vi "rsscope_core_global.vi"() -> ()   [LabVIEW 2014] (continued)
trigger search. The state search is a qualified edge search. The state search is only available for analog channel sources (Ch1 to Ch4)."}, {"Level"=4, "Class Only"=FALSE, "Identifier"="RSSCOPE_ATTR_SEARCH_TRIGGER_STATE_ENABLED", "Descriptive Name"="Search Trigger State Enabled", "Data Type"=3, "Command"="SEAR:TRIG:STAT", "Access"=2, "Range Table"="", "Read Callback"="rsscope_FormatSearchNameBoolean_ReadCallback.vi", "Write Callback"="rsscope_FormatSearchNameBoolean_WriteCallback.vi", "Supported Models"="", "Instrument Options"="", "Flags"=0, "Help"="Includes the search conditions for the state trigger event type in the next search.\n\nAvailable Repeated Capabilities:\nNone\n\nRemote-control command(s):\nSEARch:TRIGger:STATe[:STATe]"}, {"Level"=4, "Class Only"=FALSE, "Identifier"="RSSCOPE_ATTR_SEARCH_TRIGGER_STATE_CLOCK_SOURCE", "Descriptive Name"="Search Trigger State Clock Source", "Data Type"=0, "Command"="SEAR:TRIG:STAT:CSO", "Access"=2, "Range Table"="RsScope_rngSearchTriggerStateClockSource", "Read Callback"="rsscope_FormatSearchNameInt32_ReadCallback.vi", "Write Callback"="rsscope_FormatSearchNameInt32_WriteCallback.vi", "Supported Models"="", "Instrument Options"="", "Flags"=0, "Help"="Sets the source of the clock signal.\n\nAvailable Repeated Capabilities:\nNone\n\nRemote-control command(s):\nSEARch:TRIGger:STATe:CSOurce"}, {"Level"=4, "Class Only"=FALSE, "Identifier"="RSSCOPE_ATTR_SEARCH_TRIGGER_STATE_LEVEL", "Descriptive Name"="Search Trigger State Level", "Data Type"=1, "Command"="SEAR:TRIG:STAT:CLEV", "Access"=2, "Range Table"="RsScope_rngSearchTriggerClockLevel", "Read Callback"="rsscope_FormatSearchNameReal64_ReadCallback.vi", "Write Callback"="rsscope_FormatSearchNameReal64_WriteCallback.vi", "Supported Models"="", "Instrument Options"="", "Flags"=0, "Help"="Sets the trigger level of the clock signal.\n\nAvailable Repeated Capabilities:\nNone\n\nRemote-control command(s):\nSEARch:TRIGger:STATe:CLEVel"}, {"Level"=4, "Class Only"=FALSE, "Identifier"="RSSCOPE_ATTR_SEARCH_TRIGGER_STATE_CLOCK_EDGE", "Descriptive Name"="Search Trigger State Clock Edge", "Data Type"=0, "Command"="SEAR:TRIG:STAT:CEDG", "Access"=2, "Range Table"="rsscope_rngTriggerSlope", "Read Callback"="rsscope_FormatSearchNameInt32_ReadCallback.vi", "Write Callback"="rsscope_FormatSearchNameInt32_WriteCallback.vi", "Supported Models"="", "Instrument Options"="", "Flags"=0, "Help"="Sets the trigger edge of the clock signal.\n\nAvailable Repeated Capabilities:\nNone\n\nRemote-control command(s):\nSEARch:TRIGger:STATe:CEDGe"}, {"Level"=4, "Class Only"=FALSE, "Identifier"="RSSCOPE_ATTR_SEARCH_TRIGGER_STATE_COPY_FROM_A", "Descriptive Name"="Search Trigger State Copy From A", "Data Type"=4, "Command"="SEAR:TRIG:STAT:ACOP", "Access"=1, "Range Table"="", "Read Callback"="", "Write Callback"="rsscope_FormatSearchNameEvent_WriteCallback.vi", "Supported Models"="", "Instrument Options"="", "Flags"=0, "Help"="Copies the trigger event configuration from Trigger A for the selected channel source to the search condition settings. Set the selected search name with RSSCOPE_ATTR_SELECTED_SEARCH_NAME.\n\nAvailable Repeated Capabilities:\nNone\n\nRemote-control command(s):\nSEARch:TRIGger:STATe:ACOPy"}, {"Level"=4, "Class Only"=TRUE, "Identifier"="", "Descriptive Name"="Trigger Qualification", "Data Type"=0, "Command"="", "Access"=0, "Range Table"="", "Read Callback"="", "Write Callback"="", "Supported Models"="", "Instrument Options"="", "Flags"=0, "Help"="By qualifying a trigger event, you can logically combine the trigger signal with the state of other digital channel signals.\nThe instrument triggers if both of the following apply:\n- The basic conditions of the trigger event definition are fulfilled.\n- The logical conditions of the trigger qualification are true.\n\nQualification is not supported with slew rate, Data2Clock, and serial pattern trigger types.\n\nThe A-event and B-event in a trigger sequence can have their own trigger qualification. Qualification is not available for R-events (Suffix m = 3).\n\nExample: Trigger on write access of a specific device of a bus system In circuits using SPI, several slave devices use the same lines for reading and writing data, and each slave has its own select line. To trigger on write access of specific slave, the write line is the trigger source and the select line of the slave is set as qualifiying."}, {"Level"=5, "Class Only"=FALSE, "Identifier"="RSSCOPE_ATTR_SEARCH_STATE_TRIGGER_QUALIFICATION_ENABLED_CHANNEL_1", "Descriptive Name"="Search State Trigger Qualification Enabled Channel 1", "Data Type"=3, "Command"="SEAR:TRIG:STAT:A", "Access"=2, "Range Table"="", "Read Callback"="rsscope_FormatSearchNameBoolean_ReadCallback.vi", "Write Callback"="rsscope_FormatSearchNameBoolean_WriteCallback.vi", "Supported Models"="", "Instrument Options"="", "Flags"=0, "Help"="Enables the channel to be considered in the state search. You can enable all channel signals except for the trigger source. Digital channels are not available.\n\nAvailable Repeated Capabilities:\nNone\n\nRemote-control command(s):\nSEARch:TRIGger:STATe:A[:ENABle]"}, {"Level"=5, "Class Only"=FALSE, "Identifier"="RSSCOPE_ATTR_SEARCH_STATE_TRIGGER_QUALIFICATION_ENABLED_CHANNEL_2", "Descriptive Name"="Search State Trigger Qualification Enabled Channel 2", "Data Type"=3, "Command"="SEAR:TRIG:STAT:B", "Access"=2, "Range Table"="", "Read Callback"="rsscope_FormatSearchNameBoolean_ReadCallback.vi", "Write Callback"="rsscope_FormatSearchNameBoolean_WriteCallback.vi", "Supported Models"="", "Instrument Options"="", "Flags"=0, "Help"="Enables the channel to be considered in the state search. You can enable all channel signals except for the trigger source. Digital channels are not available.\n\nAvailable Repeated Capabilities:\nNone\n\nRemote-control command(s):\nSEARch:TRIGger:STATe:B[:ENABle]"}, {"Level"=5, "Class Only"=FALSE, "Identifier"="RSSCOPE_ATTR_SEARCH_STATE_TRIGGER_QUALIFICATION_ENABLED_CHANNEL_3", "Descriptive Name"="Search State Trigger Qualification Enabled Channel 3", "Data Type"=3, "Command"="SEAR:TRIG:STAT:C", "Access"=2, "Range Table"="", "Read Callback"="rsscope_FormatSearchNameBoolean_ReadCallback.vi", "Write Callback"="rsscope_FormatSearchNameBoolean_WriteCallback.vi", "Supported Models"="", "Instrument Options"="", "Flags"=0, "Help"="Enables the channel to be considered in the state search. You can enable all channel signals except for the trigger source. Digital channels are not available.\n\nAvailable Repeated Capabilities:\nNone\n\nRemote-control command(s):\nSEARch:TRIGger:STATe:C[:ENABle]"}, {"Level"=5, "Class Only"=FALSE, "Identifier"="RSSCOPE_ATTR_SEARCH_STATE_TRIGGER_QUALIFICATION_ENABLED_CHANNEL_4", "Descriptive Name"="Search State Trigger Qualification Enabled Channel 4", "Data Type"=3, "Command"="SEAR:TRIG:STAT:D", "Access"=2, "Range Table"="", "Read Callback"="rsscope_FormatSearchNameBoolean_ReadCallback.vi", "Write Callback"="rsscope_FormatSearchNameBoolean_WriteCallback.vi", "Supported Models"="", "Instrument Options"="", "Flags"=0, "Help"="Enables the channel to be considered in the state search. You can enable all channel signals except for the trigger source. Digital channels are not available.\n\nAvailable Repeated Capabilities:\nNone\n\nRemote-control command(s):\nSEARch:TRIGger:STATe:D[:ENABle]"}, {"Level"=5, "Class Only"=FALSE, "Identifier"="RSSCOPE_ATTR_SEARCH_STATE_TRIGGER_QUALIFICATION_LOGIC_CHANNEL_1", "Descriptive Name"="Search State Trigger Qualification Logic Channel 1", "Data Type"=0, "Command"="SEAR:TRIG:STAT:A:LOG", "Access"=2, "Range Table"="rsscope_rngTriggerQualificationLogic", "Read Callback"="rsscope_FormatSearchNameInt32_ReadCallback.vi", "Write Callback"="rsscope_FormatSearchNameInt32_WriteCallback.vi", "Supported Models"="", "Instrument Options"="", "Flags"=0, "Help"="Defines the logic for the indicated channel.\n\nAvailable Repeated Capabilities:\nNone\n\nRemote-control command(s):\nSEARch:TRIGger:STATe:A:LOGic"}, {"Level"=5, "Class Only"=FALSE, "Identifier"="RSSCOPE_ATTR_SEARCH_STATE_TRIGGER_QUALIFICATION_LOGIC_CHANNEL_2", "Descriptive Name"="Search State Trigger Qualification Logic Channel 2", "Data Type"=0, "Command"="SEAR:TRIG:STAT:B:LOG", "Access"=2, "Range Table"="rsscope_rngTriggerQualificationLogic", "Read Callback"="rsscope_FormatSearchNameInt32_ReadCallback.vi", "Write Callback"="rsscope_FormatSearchNameInt32_WriteCallback.vi", "Supported Models"="", "Instrument Options"="", "Flags"=0, "Help"="Defines the logic for the indicated channel.\n\nAvailable Repeated Capabilities:\nNone\n\nRemote-control command(s):\nSEARch:TRIGger:STATe:B:LOGic"}, {"Level"=5, "Class Only"=FALSE, "Identifier"="RSSCOPE_ATTR_SEARCH_STATE_TRIGGER_QUALIFICATION_LOGIC_CHANNEL_3", "Descriptive Name"="Search State Trigger Qualification Logic Channel 3", "Data Type"=0, "Command"="SEAR:TRIG:STAT:C:LOG", "Access"=2, "Range Table"="rsscope_rngTriggerQualificationLogic", "Read Callback"="rsscope_FormatSearchNameInt32_ReadCallback.vi", "Write Callback"="rsscope_FormatSearchNameInt32_WriteCallback.vi", "Supported Models"="", "Instrument Options"="", "Flags"=0, "Help"="Defines the logic for the indicated channel.\n\nAvailable Repeated Capabilities:\nNone\n\nRemote-control command(s):\nSEARch:TRIGger:STATe:C:LOGic"}, {"Level"=5, "Class Only"=FALSE, "Identifier"="RSSCOPE_ATTR_SEARCH_STATE_TRIGGER_QUALIFICATION_LOGIC_CHANNEL_4", "Descriptive Name"="Search State Trigger Qualification Logic Channel 4", "Data Type"=0, "Command"="SEAR:TRIG:STAT:D:LOG", "Access"=2, "Range Table"="rsscope_rngTriggerQualificationLogic", "Read Callback"="rsscope_FormatSearchNameInt32_ReadCallback.vi", "Write Callback"="rsscope_FormatSearchNameInt32_WriteCallback.vi", "Supported Models"="", "Instrument Options"="", "Flags"=0, "Help"="Defines the logic for the indicated channel.\n\nAvailable Repeated Capabilities:\nNone\n\nRemote-control command(s):\nSEARch:TRIGger:STATe:D:LOGic"}, {"Level"=5, "Class Only"=FALSE, "Identifier"="RSSCOPE_ATTR_SEARCH_STATE_TRIGGER_QUALIFICATION_LOGIC_CHANNELS_1_2", "Descriptive Name"="Search State Trigger Qualification Logic Channels 1 2", "Data Type"=0, "Command"="SEAR:TRIG:STAT:AB:LOG", "Access"=2, "Range Table"="rsscope_rngLogic", "Read Callback"="rsscope_FormatSearchNameInt32_ReadCallback.vi", "Write Callback"="rsscope_FormatSearchNameInt32_WriteCallback.vi", "Supported Models"="", "Instrument Options"="", "Flags"=0, "Help"="Defines the logical combination of the indicated channels after evaluating the previous logical operations.\n\nAvailable Repeated Capabilities:\nNone\n\nRemote-control command(s):\nSEARch:TRIGger:STATe:AB:LOGic"}, {"Level"=5, "Class Only"=FALSE, "Identifier"="RSSCOPE_ATTR_SEARCH_STATE_TRIGGER_QUALIFICATION_LOGIC_CHANNELS_3_4", "Descriptive Name"="Search State Trigger Qualification Logic Channels 3 4", "Data Type"=0, "Command"="SEAR:TRIG:STAT:CD:LOG", "Access"=2, "Range Table"="rsscope_rngLogic", "Read Callback"="rsscope_FormatSearchNameInt32_ReadCallback.vi", "Write Callback"="rsscope_FormatSearchNameInt32_WriteCallback.vi", "Supported Models"="", "Instrument Options"="", "Flags"=0, "Help"="Defines the logical combination of the indicated channels after evaluating the previous logical operations.\n\nAvailable Repeated Capabilities:\nNone\n\nRemote-control command(s):\nSEARch:TRIGger:STATe:CD:LOGic"}, {"Level"=5, "Class Only"=FALSE, "Identifier"="RSSCOPE_ATTR_SEARCH_STATE_TRIGGER_QUALIFICATION_LOGIC_CHANNELS_ALL", "Descriptive Name"="Search State Trigger Qualification Logic Channels All", "Data Type"=0, "Command"="SEAR:TRIG:STAT:ABCD:LOG", "Access"=2, "Range Table"="rsscope_rngLogic", "Read Callback"="rsscope_FormatSearchNameInt32_ReadCallback.vi", "Write Callback"="rsscope_FormatSearchNameInt32_WriteCallback.vi", "Supported Models"="", "Instrument Options"="", "Flags"=0, "Help"="Defines the logical combination of the indicated channels after evaluating the result of channels 1+2 and 3+4.\n\nAvailable Repeated Capabilities:\nNone\n\nRemote-control command(s):\nSEARch:TRIGger:STATe:ABCD:LOGic"}, {"Level"=3, "Class Only"=TRUE, "Identifier"="", "Descriptive Name"="Pattern", "Data Type"=0, "Command"="", "Access"=0, "Range Table"="", "Read Callback"="", "Write Callback"="", "Supported Models"="", "Instrument Options"="", "Flags"=0, "Help"="This class configures the conditions for the pattern trigger search."}, {"Level"=4, "Class Only"=FALSE, "Identifier"="RSSCOPE_ATTR_SEARCH_TRIGGER_PATTERN_ENABLED", "Descriptive Name"="Search Trigger Pattern Enabled", "Data Type"=3, "Command"="SEAR:TRIG:PATT", "Access"=2, "Range Table"="", "Read Callback"="rsscope_FormatSearchNameBoolean_ReadCallback.vi", "Write Callback"="rsscope_FormatSearchNameBoolean_WriteCallback.vi", "Supported Models"="", "Instrument Options"="", "Flags"=0, "Help"="Includes the search conditions for the pattern trigger event type in the next search.\n\nAvailable Repeated Capabilities:\nNone\n\nRemote-control command(s):\nSEARch:TRIGger:PATTern[:STATe]"}, {"Level"=4, "Class Only"=FALSE, "Identifier"="RSSCOPE_ATTR_SEARCH_TRIGGER_PATTERN_MODE", "Descriptive Name"="Search Trigger Pattern Mode", "Data Type"=0, "Command"="SEAR:TRIG:PATT:MODE", "Access"=2, "Range Table"="RsScope_rngSearchTriggerPatternMode", "Read Callback"="rsscope_FormatSearchNameInt32_ReadCallback.vi", "Write Callback"="rsscope_FormatSearchNameInt32_WriteCallback.vi", "Supported Models"="", "Instrument Options"="", "Flags"=0, "Help"="Adds additional time limitation to the pattern definition.\n\nAvailable Repeated Capabilities:\nNone\n\nRemote-control command(s):\nSEARch:TRIGger:PATTern:MODE"}, {"Level"=4, "Class Only"=FALSE, "Identifier"="RSSCOPE_ATTR_SEARCH_TRIGGER_PATTERN_TIMEOUT_CONDITION", "Descriptive Name"="Search Trigger Pattern Timeout Condition", "Data Type"=0, "Command"="SEAR:TRIG:PATT:TIM:MODE", "Access"=2, "Range Table"="RsScope_rngSearchTriggerPatternTimeoutMode", "Read Callback"="rsscope_FormatSearchNameInt32_ReadCallback.vi", "Write Callback"="rsscope_FormatSearchNameInt32_WriteCallback.vi", "Supported Models"="", "Instrument Options"="", "Flags"=0, "Help"="Defines the condition for the timeout.\n\nAvailable Repeated Capabilities:\nNone\n\nRemote-control command(s):\nSEARch:TRIGger:PATTern:TIMeout:MODE"}, {"Level"=4, "Class Only"=FALSE, "Identifier"="RSSCOPE_ATTR_SEARCH_TRIGGER_PATTERN_TIMEOUT", "Descriptive Name"="Search Trigger Pattern Timeout", "Data Type"=1, "Command"="SEAR:TRIG:PATT:TIM", "Access"=2, "Range Table"="RsScope_rngSearchTriggerWidth", "Read Callback"="rsscope_FormatSearchNameReal64_ReadCallback.vi", "Write Callback"="rsscope_FormatSearchNameReal64_WriteCallback.vi", "Supported Models"="", "Instrument Options"="", "Flags"=0, "Help"="Defines how long the result of the pattern condition must keep the given state.\n\nAvailable Repeated Capabilities:\nNone\n\nRemote-control command(s):\nSEARch:TRIGger:PATTern:TIMeout[:TIME]"}, {"Level"=4, "Class Only"=FALSE, "Identifier"="RSSCOPE_ATTR_SEARCH_TRIGGER_PATTERN_WIDTH", "Descriptive Name"="Search Trigger Pattern Width", "Data Type"=1, "Command"="SEAR:TRIG:PATT:WIDT", "Access"=2, "Range Table"="RsScope_rngSearchTriggerWidth", "Read Callback"="rsscope_FormatSearchNameReal64_ReadCallback.vi", "Write Callback"="rsscope_FormatSearchNameReal64_WriteCallback.vi", "Supported Models"="", "Instrument Options"="", "Flags"=0, "Help"="For the ranges &apos;Within&apos; and &apos;Outside&apos;, the width defines the center of a range which is defined by the limits &apos;Delta&apos;.\nFor the ranges &apos;Shorter&apos; and &apos;Longer&apos;, the width defines the maximum and minimum pulse width, respectively.\n\nAvailable Repeated Capabilities:\nNone\n\nRemote-control command(s):\nSEARch:TRIGger:PATTern:WIDTh[:WIDTh]"}, {"Level"=4, "Class Only"=FALSE, "Identifier"="RSSCOPE_ATTR_SEARCH_TRIGGER_PATTERN_WIDTH_DELTA", "Descriptive Name"="Search Trigger Pattern Width Delta", "Data Type"=1, "Command"="SEAR:TRIG:PATT:WIDT:DELT", "Access"=2, "Range Table"="RsScope_rngSearchTriggerPatternDelta", "Read Callback"="rsscope_FormatSearchNameReal64_ReadCallback.vi", "Write Callback"="rsscope_FormatSearchNameReal64_WriteCallback.vi", "Supported Models"="", "Instrument Options"="", "Flags"=0, "Help"="For the ranges &apos;Within&apos; and &apos;Outside&apos;, the width defines the center of a range which is defined by the limits &apos;+/-Delta&apos;. For the ranges &apos;Shorter&apos; and &apos;Longer&apos;, the width defines the maximum and minimum pulse width, respectively.\n\nAvailable Repeated Capabilities:\nNone\n\nRemote-control command(s):\nSEARch:TRIGger:PATTern:WIDTh:DELTa"}, {"Level"=4, "Class Only"=FALSE, "Identifier"="RSSCOPE_ATTR_SEARCH_TRIGGER_PATTERN_WIDTH_CONDITION", "Descriptive Name"="Search Trigger Pattern Width Condition", "Data Type"=0, "Command"="SEAR:TRIG:PATT:WIDT:RANG", "Access"=2, "Range Table"="rsscope_rngWidthCondition", "Read Callback"="rsscope_FormatSearchNameInt32_ReadCallback.vi", "Write Callback"="rsscope_FormatSearchNameInt32_WriteCallback.vi", "Supported Models"="", "Instrument Options"="", "Flags"=0, "Help"="Defines how the range of a pulse width is defined for keeping up the true result of the pattern condition.\n\nAvailable Repeated Capabilities:\nNone\n\nRemote-control command(s):\nSEARch:TRIGger:PATTern:WIDTh:RANGe"}, {"Level"=4, "Class Only"=FALSE, "Identifier"="RSSCOPE_ATTR_SEARCH_TRIGGER_PATTERN_COPY_FROM_A", "Descriptive Name"="Search Trigger Pattern Copy From A", "Data Type"=4, "Command"="SEAR:TRIG:PATT:ACOP", "Access"=1, "Range Table"="", "Read Callback"="", "Write Callback"="rsscope_FormatSearchNameEvent_WriteCallback.vi", "Supported Models"="", "Instrument Options"="", "Flags"=0, "Help"="Copies the trigger event configuration from Trigger A for the selected channel source to the search condition settings. Set the selected search name with RSSCOPE_ATTR_SELECTED_SEARCH_NAME.\n\nAvailable Repeated Capabilities:\nNone\n\nRemote-control command(s):\nSEARch:TRIGger:PATTern:ACOPy"}, {"Level"=4, "Class Only"=TRUE, "Identifier"="", "Descriptive Name"="Trigger Qualification", "Data Type"=0, "Command"="", "Access"=0, "Range Table"="", "Read Callback"="", "Write Callback"="", "Supported Models"="", "Instrument Options"="", "Flags"=0, "Help"="By qualifying a trigger event, you can logically combine the trigger signal with the state of other digital channel signals.\nThe instrument triggers if both of the following apply:\n- The basic conditions of the trigger event definition are fulfilled.\n- The logical conditions of the trigger qualification are true.\n\nQualification is not supported with slew rate, Data2Clock, and serial pattern trigger types.\n\nThe A-event and B-event in a trigger sequence can have their own trigger qualification. Qualification is not available for R-events (Suffix m = 3).\n\nExample: Trigger on write access of a specific device of a bus system In circuits using SPI, several slave devices use the same lines for reading and writing data, and each slave has its own select line. To trigger on write access of specific slave, the write line is the trigger source and the select line of the slave is set as qualifiying."}, {"Level"=5, "Class Only"=FALSE, "Identifier"="RSSCOPE_ATTR_SEARCH_PATTERN_TRIGGER_QUALIFICATION_ENABLED_CHANNEL_1", "Descriptive Name"="Search Pattern Trigger Qualification Enabled Channel 1", "Data Type"=3, "Command"="SEAR:TRIG:PATT:A", "Access"=2, "Range Table"="", "Read Callback"="rsscope_FormatSearchNameBoolean_ReadCallback.vi", "Write Callback"="rsscope_FormatSearchNameBoolean_WriteCallback.vi", "Supported Models"="", "Instrument Options"="", "Flags"=0, "Help"="Enables the channel to be considered in the pattern search. The trigger source channel is selected by default. Digital channels are not available.\n\nAvailable Repeated Capabilities:\nNone\n\nRemote-control command(s):\nSEARch:TRIGger:PATTern:A[:ENABle]"}, {"Level"=5, "Class Only"=FALSE, "Identifier"="RSSCOPE_ATTR_SEARCH_PATTERN_TRIGGER_QUALIFICATION_ENABLED_CHANNEL_2", "Descriptive Name"="Search Pattern Trigger Qualification Enabled Channel 2", "Data Type"=3, "Command"="SEAR:TRIG:PATT:B", "Access"=2, "Range Table"="", "Read Callback"="rsscope_FormatSearchNameBoolean_ReadCallback.vi", "Write Callback"="rsscope_FormatSearchNameBoolean_WriteCallback.vi", "Supported Models"="", "Instrument Options"="", "Flags"=0, "Help"="Enables the channel to be considered in the pattern search. The trigger source channel is selected by default. Digital channels are not available.\n\nAvailable Repeated Capabilities:\nNone\n\nRemote-control command(s):\nSEARch:TRIGger:PATTern:B[:ENABle]"}, {"Level"=5, "Class Only"=FALSE, "Identifier"="RSSCOPE_ATTR_SEARCH_PATTERN_TRIGGER_QUALIFICATION_ENABLED_CHANNEL_3", "Descriptive Name"="Search Pattern Trigger Qualification Enabled Channel 3", "Data Type"=3, "Command"="SEAR:TRIG:PATT:C", "Access"=2, "Range Table"="", "Read Callback"="rsscope_FormatSearchNameBoolean_ReadCallback.vi", "Write Callback"="rsscope_FormatSearchNameBoolean_WriteCallback.vi", "Supported Models"="", "Instrument Options"="", "Flags"=0, "Help"="Enables the channel to be considered in the pattern search. The trigger source channel is selected by default. Digital channels are not available.\n\nAvailable Repeated Capabilities:\nNone\n\nRemote-control command(s):\nSEARch:TRIGger:PATTern:C[:ENABle]"}, {"Level"=5, "Class Only"=FALSE, "Identifier"="RSSCOPE_ATTR_SEARCH_PATTERN_TRIGGER_QUALIFICATION_ENABLED_CHANNEL_4", "Descriptive Name"="Search Pattern Trigger Qualification Enabled Channel 4", "Data Type"=3, "Command"="SEAR:TRIG:PATT:D", "Access"=2, "Range Table"="", "Read Callback"="rsscope_FormatSearchNameBoolean_ReadCallback.vi", "Write Callback"="rsscope_FormatSearchNameBoolean_WriteCallback.vi", "Supported Models"="", "Instrument Options"="", "Flags"=0, "Help"="Enables the channel to be considered in the pattern search. The trigger source channel is selected by default. Digital channels are not available.\n\nAvailable Repeated Capabilities:\nNone\n\nRemote-control command(s):\nSEARch:TRIGger:PATTern:D[:ENABle]"}, {"Level"=5, "Class Only"=FALSE, "Identifier"="RSSCOPE_ATTR_SEARCH_PATTERN_TRIGGER_QUALIFICATION_LOGIC_CHANNEL_1", "Descriptive Name"="Search Pattern Trigger Qualification Logic Channel 1", "Data Type"=0, "Command"="SEAR:TRIG:PATT:A:LOG", "Access"=2, "Range Table"="rsscope_rngTriggerQualificationLogic", "Read Callback"="rsscope_FormatSearchNameInt32_ReadCallback.vi", "Write Callback"="rsscope_FormatSearchNameInt32_WriteCallback.vi", "Supported Models"="", "Instrument Options"="", "Flags"=0, "Help"="Defines the logic for the indicated channel.\n\nAvailable Repeated Capabilities:\nNone\n\nRemote-control command(s):\nSEARch:TRIGger:PATTern:A:LOGic"}, {"Level"=5, "Class Only"=FALSE, "Identifier"="RSSCOPE_ATTR_SEARCH_PATTERN_TRIGGER_QUALIFICATION_LOGIC_CHANNEL_2", "Descriptive Name"="Search Pattern Trigger Qualification Logic Channel 2", "Data Type"=0, "Command"="SEAR:TRIG:PATT:B:LOG", "Access"=2, "Range Table"="rsscope_rngTriggerQualificationLogic", "Read Callback"="rsscope_FormatSearchNameInt32_ReadCallback.vi", "Write Callback"="rsscope_FormatSearchNameInt32_WriteCallback.vi", "Supported Models"="", "Instrument Options"="", "Flags"=0, "Help"="Defines the logic for the indicated channel.\n\nAvailable Repeated Capabilities:\nNone\n\nRemote-control command(s):\nSEARch:TRIGger:PATTern:B:LOGic"}, {"Level"=5, "Class Only"=FALSE, "Identifier"="RSSCOPE_ATTR_SEARCH_PATTERN_TRIGGER_QUALIFICATION_LOGIC_CHANNEL_3", "Descriptive Name"="Search Pattern Trigger Qualification Logic Channel 3", "Data Type"=0, "Command"="SEAR:TRIG:PATT:C:LOG", "Access"=2, "Range Table"="rsscope_rngTriggerQualificationLogic", "Read Callback"="rsscope_FormatSearchNameInt32_ReadCallback.vi", "Write Callback"="rsscope_FormatSearchNameInt32_WriteCallback.vi", "Supported Models"="", "Instrument Options"="", "Flags"=0, "Help"="Defines the logic for the indicated channel.\n\nAvailable Repeated Capabilities:\nNone\n\nRemote-control command(s):\nSEARch:TRIGger:PATTern:C:LOGic"}, {"Level"=5, "Class Only"=FALSE, "Identifier"="RSSCOPE_ATTR_SEARCH_PATTERN_TRIGGER_QUALIFICATION_LOGIC_CHANNEL_4", "Descriptive Name"="Search Pattern Trigger Qualification Logic Channel 4", "Data Type"=0, "Command"="SEAR:TRIG:PATT:D:LOG", "Access"=2, "Range Table"="rsscope_rngTriggerQualificationLogic", "Read Callback"="rsscope_FormatSearchNameInt32_ReadCallback.vi", "Write Callback"="rsscope_FormatSearchNameInt32_WriteCallback.vi", "Supported Models"="", "Instrument Options"="", "Flags"=0, "Help"="Defines the logic for the indicated channel.\n\nAvailable Repeated Capabilities:\nNone\n\nRemote-control command(s):\nSEARch:TRIGger:PATTern:D:LOGic"}, {"Level"=5, "Class Only"=FALSE, "Identifier"="RSSCOPE_ATTR_SEARCH_PATTERN_TRIGGER_QUALIFICATION_LOGIC_CHANNELS_1_2", "Descriptive Name"="Search Pattern Trigger Qualification Logic Channels 1 2", "Data Type"=0, "Command"="SEAR:TRIG:PATT:AB:LOG", "Access"=2, "Range Table"="rsscope_rngLogic", "Read Callback"="rsscope_FormatSearchNameInt32_ReadCallback.vi", "Write Callback"="rsscope_FormatSearchNameInt32_WriteCallback.vi", "Supported Models"="", "Instrument Options"="", "Flags"=0, "Help"="Defines the logical combination of the indicated channels after evaluating the previous logical operations.\n\nAvailable Repeated Capabilities:\nNone\n\nRemote-control command(s):\nSEARch:TRIGger:PATTern:AB:LOGic"}, {"Level"=5, "Class Only"=FALSE, "Identifier"="RSSCOPE_ATTR_SEARCH_PATTERN_TRIGGER_QUALIFICATION_LOGIC_CHANNELS_3_4", "Descriptive Name"="Search Pattern Trigger Qualification Logic Channels 3 4", "Data Type"=0, "Command"="SEAR:TRIG:PATT:CD:LOG", "Access"=2, "Range Table"="rsscope_rngLogic", "Read Callback"="rsscope_FormatSearchNameInt32_ReadCallback.vi", "Write Callback"="rsscope_FormatSearchNameInt32_WriteCallback.vi", "Supported Models"="", "Instrument Options"="", "Flags"=0, "Help"="Defines the logical combination of the indicated channels after evaluating the previous logical operations.\n\nAvailable Repeated Capabilities:\nNone\n\nRemote-control command(s):\nSEARch:TRIGger:PATTern:CD:LOGic"}, {"Level"=5, "Class Only"=FALSE, "Identifier"="RSSCOPE_ATTR_SEARCH_PATTERN_TRIGGER_QUALIFICATION_LOGIC_CHANNELS_ALL", "Descriptive Name"="Search Pattern Trigger Qualification Logic Channels All", "Data Type"=0, "Command"="SEAR:TRIG:PATT:ABCD:LOG", "Access"=2, "Range Table"="rsscope_rngLogic", "Read Callback"="rsscope_FormatSearchNameInt32_ReadCallback.vi", "Write Callback"="rsscope_FormatSearchNameInt32_WriteCallback.vi", "Supported Models"="", "Instrument Options"="", "Flags"=0, "Help"="Defines the logical combination of the indicated channels after evaluating the result of channels 1+2 and 3+4.\n\nAvailable Repeated Capabilities:\nNone\n\nRemote-control command(s):\nSEARch:TRIGger:PATTern:ABCD:LOGic"}, {"Level"=2, "Class Only"=TRUE, "Identifier"="", "Descriptive Name"="Scope", "Data Type"=0, "Command"="", "Access"=0, "Range Table"="", "Read Callback"="", "Write Callback"="", "Supported Models"="", "Instrument Options"="", "Flags"=0, "Help"="Defines the Search scope."}, {"Level"=3, "Class Only"=FALSE, "Identifier"="RSSCOPE_ATTR_SEARCH_GATE_ENABLED", "Descriptive Name"="Search Gate Enabled", "Data Type"=3, "Command"="SEAR:GATE", "Access"=2, "Range Table"="", "Read Callback"="rsscope_FormatSearchNameBoolean_ReadCallback.vi", "Write Callback"="rsscope_FormatSearchNameBoolean_WriteCallback.vi", "Supported Models"="", "Instrument Options"="", "Flags"=0, "Help"="Performs the search only on the defined gate area of the source waveform.\n\nAvailable Repeated Capabilities:\nNone\n\nRemote-control command(s):\nSEARch:GATE[:STATe]"}, {"Level"=3, "Class Only"=FALSE, "Identifier"="RSSCOPE_ATTR_SEARCH_GATE_SHOW", "Descriptive Name"="Search Gate Show", "Data Type"=3, "Command"="SEAR:GATE:SHOW", "Access"=2, "Range Table"="", "Read Callback"="rsscope_FormatSearchNameBoolean_ReadCallback.vi", "Write Callback"="rsscope_FormatSearchNameBoolean_WriteCallback.vi", "Supported Models"="", "Instrument Options"="", "Flags"=0, "Help"="If enabled, the gate area is indicated in the source diagram.\n\nAvailable Repeated Capabilities:\nNone\n\nRemote-control command(s):\nSEARch:GATE:SHOW"}, {"Level"=3, "Class Only"=FALSE, "Identifier"="RSSCOPE_ATTR_ZOOM_COUPLING", "Descriptive Name"="Zoom Coupling", "Data Type"=3, "Command"="SEAR:GATE:ZCO", "Access"=2, "Range Table"="", "Read Callback"="rsscope_FormatSearchNameBoolean_ReadCallback.vi", "Write Callback"="rsscope_FormatSearchNameBoolean_WriteCallback.vi", "Supported Models"="", "Instrument Options"="", "Flags"=0, "Help"="If enabled, the gate area is set to the limits of a zoom area.\n\nAvailable Repeated Capabilities:\nNone\n\nRemote-control command(s):\nSEARch:GATE:ZCOupling"}, {"Level"=3, "Class Only"=FALSE, "Identifier"="RSSCOPE_ATTR_SEARCH_GATE_MODE", "Descriptive Name"="Search Gate Mode", "Data Type"=0, "Command"="SEAR:GATE:MODE", "Access"=2, "Range Table"="rsscope_rngAbsRel", "Read Callback"="rsscope_FormatSearchNameInt32_ReadCallback.vi", "Write Callback"="rsscope_FormatSearchNameInt32_WriteCallback.vi", "Supported Models"="", "Instrument Options"="", "Flags"=0, "Help"="Defines whether the gate settings are configured using absolute or relative values.\n\nAvailable Repeated Capabilities:\nNone\n\nRemote-control command(s):\nSEARch:GATE:MODE"}, {"Level"=3, "Class Only"=FALSE, "Identifier"="RSSCOPE_ATTR_SEARCH_GATE_ABSOLUTE_START", "Descriptive Name"="Search Gate Absolute Start", "Data Type"=1, "Command"="SEAR:GATE:ABS:STAR", "Access"=2, "Range Table"="", "Read Callback"="rsscope_FormatSearchNameReal64_ReadCallback.vi", "Write Callback"="rsscope_FormatSearchNameReal64_WriteCallback.vi", "Supported Models"="", "Instrument Options"="", "Flags"=0, "Help"="Defines the starting value for the gate.\n\nAvailable Repeated Capabilities:\nNone\n\nRemote-control command(s):\nSEARch:GATE:ABSolute:STARt"}, {"Level"=3, "Class Only"=FALSE, "Identifier"="RSSCOPE_ATTR_SEARCH_GATE_RELATIVE_START", "Descriptive Name"="Search Gate Relative Start", "Data Type"=1, "Command"="SEAR:GATE:REL:STAR", "Access"=2, "Range Table"="", "Read Callback"="rsscope_FormatSearchNameReal64_ReadCallback.vi", "Write Callback"="rsscope_FormatSearchNameReal64_WriteCallback.vi", "Supported Models"="", "Instrument Options"="", "Flags"=0, "Help"="Defines the starting value for the gate.\n\nAvailable Repeated Capabilities:\nNone\n\nRemote-control command(s):\nSEARch:GATE:RELative:STARt"}, {"Level"=3, "Class Only"=FALSE, "Identifier"="RSSCOPE_ATTR_SEARCH_GATE_ABSOLUTE_STOP", "Descriptive Name"="Search Gate Absolute Stop", "Data Type"=1, "Command"="SEAR:GATE:ABS:STOP", "Access"=2, "Range Table"="", "Read Callback"="rsscope_FormatSearchNameReal64_ReadCallback.vi", "Write Callback"="rsscope_FormatSearchNameReal64_WriteCallback.vi", "Supported Models"="", "Instrument Options"="", "Flags"=0, "Help"="Defines the end value for the gate.\n\nAvailable Repeated Capabilities:\nNone\n\nRemote-control command(s):\nSEARch:GATE:ABSolute:STOP"}, {"Level"=3, "Class Only"=FALSE, "Identifier"="RSSCOPE_ATTR_SEARCH_GATE_RELATIVE_STOP", "Descriptive Name"="Search Gate Relative Stop", "Data Type"=1, "Command"="SEAR:GATE:REL:STOP", "Access"=2, "Range Table"="", "Read Callback"="rsscope_FormatSearchNameReal64_ReadCallback.vi", "Write Callback"="rsscope_FormatSearchNameReal64_WriteCallback.vi", "Supported Models"="", "Instrument Options"="", "Flags"=0, "Help"="Defines the end value for the gate.\n\nAvailable Repeated Capabilities:\nNone\n\nRemote-control command(s):\nSEARch:GATE:RELative:STOP"}, {"Level"=2, "Class Only"=TRUE, "Identifier"="", "Descriptive Name"="Result Presentation", "Data Type"=0, "Command"="", "Access"=0, "Range Table"="", "Read Callback"="", "Write Callback"="", "Supported Models"="", "Instrument Options"="", "Flags"=0, "Help"="Search results are displayed in a table in the &apos;Search Results&apos; box. The result tables can be sorted by x-position or value. You can define a maximum number of table entries. In addition, a zoom window for each search result can be displayed automatically in the source diagram so that you can analyze the result in more detail."}, {"Level"=3, "Class Only"=FALSE, "Identifier"="RSSCOPE_ATTR_SEARCH_RESULT_TABLE_ENABLED", "Descriptive Name"="Search Result Table Enabled", "Data Type"=3, "Command"="SEAR:RES:SHOW", "Access"=2, "Range Table"="", "Read Callback"="rsscope_FormatSearchNameBoolean_ReadCallback.vi", "Write Callback"="rsscope_FormatSearchNameBoolean_WriteCallback.vi", "Supported Models"="", "Instrument Options"="", "Flags"=0, "Help"="Displays or hides the search result table.\n\nAvailable Repeated Capabilities:\nNone\n\nRemote-control command(s):\nSEARch:RESult:SHOW"}, {"Level"=3, "Class Only"=FALSE, "Identifier"="RSSCOPE_ATTR_SEARCH_RESULT_SORT_MODE", "Descriptive Name"="Search Result Sort Mode", "Data Type"=0, "Command"="SEAR:RES:SORT", "Access"=2, "Range Table"="RsScope_rngSearchSortMode", "Read Callback"="rsscope_FormatSearchNameInt32_ReadCallback.vi", "Write Callback"="rsscope_FormatSearchNameInt32_WriteCallback.vi", "Supported Models"="", "Instrument Options"="", "Flags"=0, "Help"="Sorts the search result table by x-value position or value of the result.\n\nAvailable Repeated Capabilities:\nNone\n\nRemote-control command(s):\nSEARch:RESult:SORT[:MODE]"}, {"Level"=3, "Class Only"=FALSE, "Identifier"="RSSCOPE_ATTR_SEARCH_RESULT_SORT_ASCENDING", "Descriptive Name"="Search Result Sort Ascending", "Data Type"=3, "Command"="SEAR:RES:SORT:ASC", "Access"=2, "Range Table"="", "Read Callback"="rsscope_FormatSearchNameBoolean_ReadCallback.vi", "Write Callback"="rsscope_FormatSearchNameBoolean_WriteCallback.vi", "Supported Models"="", "Instrument Options"="", "Flags"=0, "Help"="If enabled, the results are listed in asscending order, i.e. the smallest value at the top.\n\nAvailable Repeated Capabilities:\nNone\n\nRemote-control command(s):\nSEARch:RESult:SORT:ASCending"}, {"Level"=3, "Class Only"=FALSE, "Identifier"="RSSCOPE_ATTR_SEARCH_RESULT_MAX_COUNT", "Descriptive Name"="Search Result Max Count", "Data Type"=5, "Command"="SEAR:RES:LIM", "Access"=2, "Range Table"="RsScope_rngConfigureSearchResultMaxCount", "Read Callback"="rsscope_FormatSearchNameInt64_ReadCallback.vi", "Write Callback"="rsscope_FormatSearchNameInt64_WriteCallback.vi", "Supported Models"="", "Instrument Options"="", "Flags"=0, "Help"="Defines the maximum number of entries in the search result table.\n\nAvailable Repeated Capabilities:\nNone\n\nRemote-control command(s):\nSEARch:RESult:LIMit"}, {"Level"=3, "Class Only"=FALSE, "Identifier"="RSSCOPE_ATTR_SEARCH_RESULT_ZOOM_WINDOW", "Descriptive Name"="Search Result Zoom Window", "Data Type"=3, "Command"="SEAR:RESD:SHOW", "Access"=2, "Range Table"="", "Read Callback"="rsscope_FormatSearchNameBoolean_ReadCallback.vi", "Write Callback"="rsscope_FormatSearchNameBoolean_WriteCallback.vi", "Supported Models"="", "Instrument Options"="", "Flags"=0, "Help"="If enabled, a zoom window is displayed for the currently selected search result. The zoom area is indicated in the diagram that displays the source waveform of the search.\n\nAvailable Repeated Capabilities:\nNone\n\nRemote-control command(s):\nSEARch:RESDiagram:SHOW"}, {"Level"=3, "Class Only"=FALSE, "Identifier"="RSSCOPE_ATTR_SEARCH_RESULT_ZOOM_HORIZONTAL_MODE", "Descriptive Name"="Search Result Zoom Horizontal Mode", "Data Type"=0, "Command"="SEAR:RESD:HORZ:MODE", "Access"=2, "Range Table"="rsscope_rngAbsRel", "Read Callback"="rsscope_FormatSearchNameInt32_ReadCallback.vi", "Write Callback"="rsscope_FormatSearchNameInt32_WriteCallback.vi", "Supported Models"="", "Instrument Options"="", "Flags"=0, "Help"="Defines whether absolute or relative values are used to specify the x-axis values.\n\nAvailable Repeated Capabilities:\nNone\n\nRemote-control command(s):\nSEARch:RESDiagram:HORZ:MODE"}, {"Level"=3, "Class Only"=FALSE, "Identifier"="RSSCOPE_ATTR_SEARCH_RESULT_ZOOM_ABSOLUTE_HORIZONTAL_POSITION", "Descriptive Name"="Search Result Zoom Absolute Horizontal Position", "Data Type"=1, "Command"="SEAR:RESD:HORZ:ABS:POS", "Access"=2, "Range Table"="", "Read Callback"="rsscope_FormatSearchNameReal64_ReadCallback.vi", "Write Callback"="rsscope_FormatSearchNameReal64_WriteCallback.vi", "Supported Models"="", "Instrument Options"="", "Flags"=0, "Help"="Defines the x-value of the centerpoint of the zoom area.\n\nAvailable Repeated Capabilities:\nNone\n\nRemote-control command(s):\nSEARch:RESDiagram:HORZ:ABSolute:POSition"}, {"Level"=3, "Class Only"=FALSE, "Identifier"="RSSCOPE_ATTR_SEARCH_RESULT_ZOOM_ABSOLUTE_HORIZONTAL_RANGE", "Descriptive Name"="Search Result Zoom Absolute Horizontal Range", "Data Type"=1, "Command"="SEAR:RESD:HORZ:ABS:SPAN", "Access"=2, "Range Table"="", "Read Callback"="rsscope_FormatSearchNameReal64_ReadCallback.vi", "Write Callback"="rsscope_FormatSearchNameReal64_WriteCallback.vi", "Supported Models"="", "Instrument Options"="", "Flags"=0, "Help"="Defines the width of the zoom area.\n\nAvailable Repeated Capabilities:\nNone\n\nRemote-control command(s):\nSEARch:RESDiagram:HORZ:ABSolute:SPAN"}, {"Level"=3, "Class Only"=FALSE, "Identifier"="RSSCOPE_ATTR_SEARCH_RESULT_ZOOM_RELATIVE_HORIZONTAL_POSITION", "Descriptive Name"="Search Result Zoom Relative Horizontal Position", "Data Type"=1, "Command"="SEAR:RESD:HORZ:REL:POS", "Access"=2, "Range Table"="", "Read Callback"="rsscope_FormatSearchNameReal64_ReadCallback.vi", "Write Callback"="rsscope_FormatSearchNameReal64_WriteCallback.vi", "Supported Models"="", "Instrument Options"="", "Flags"=0, "Help"="Defines the x-value of the centerpoint of the zoom area.\n\nAvailable Repeated Capabilities:\nNone\n\nRemote-control command(s):\nSEARch:RESDiagram:HORZ:RELative:POSition"}, {"Level"=3, "Class Only"=FALSE, "Identifier"="RSSCOPE_ATTR_SEARCH_RESULT_ZOOM_RELATIVE_HORIZONTAL_RANGE", "Descriptive Name"="Search Result Zoom Relative Horizontal Range", "Data Type"=1, "Command"="SEAR:RESD:HORZ:REL:SPAN", "Access"=2, "Range Table"="", "Read Callback"="rsscope_FormatSearchNameReal64_ReadCallback.vi", "Write Callback"="rsscope_FormatSearchNameReal64_WriteCallback.vi", "Supported Models"="", "Instrument Options"="", "Flags"=0, "Help"="Defines the width of the zoom area.\n\nAvailable Repeated Capabilities:\nNone\n\nRemote-control command(s):\nSEARch:RESDiagram:HORZ:RELative:SPAN"}, {"Level"=3, "Class Only"=FALSE, "Identifier"="RSSCOPE_ATTR_SEARCH_RESULT_ZOOM_VERTICAL_MODE", "Descriptive Name"="Search Result Zoom Vertical Mode", "Data Type"=0, "Command"="SEAR:RESD:VERT:MODE", "Access"=2, "Range Table"="rsscope_rngAbsRel", "Read Callback"="rsscope_FormatSearchNameInt32_ReadCallback.vi", "Write Callback"="rsscope_FormatSearchNameInt32_WriteCallback.vi", "Supported Models"="", "Instrument Options"="", "Flags"=0, "Help"="Defines whether absolute or relative values are used to specify the y-axis values.\n\nAvailable Repeated Capabilities:\nNone\n\nRemote-control command(s):\nSEARch:RESDiagram:VERT:MODE"}, {"Level"=3, "Class Only"=FALSE, "Identifier"="RSSCOPE_ATTR_SEARCH_RESULT_ZOOM_ABSOLUTE_VERTICAL_POSITION", "Descriptive Name"="Search Result Zoom Absolute Vertical Position", "Data Type"=1, "Command"="SEAR:RESD:VERT:ABS:POS", "Access"=2, "Range Table"="", "Read Callback"="rsscope_FormatSearchNameReal64_ReadCallback.vi", "Write Callback"="rsscope_FormatSearchNameReal64_WriteCallback.vi", "Supported Models"="", "Instrument Options"="", "Flags"=0, "Help"="Defines the y-value of the centerpoint of the zoom area.\n\nAvailable Repeated Capabilities:\nNone\n\nRemote-control command(s):\nSEARch:RESDiagram:VERT:ABSolute:POSition"}, {"Level"=3, "Class Only"=FALSE, "Identifier"="RSSCOPE_ATTR_SEARCH_RESULT_ZOOM_ABSOLUTE_VERTICAL_RANGE", "Descriptive Name"="Search Result Zoom Absolute Vertical Range", "Data Type"=1, "Command"="SEAR:RESD:VERT:ABS:SPAN", "Access"=2, "Range Table"="", "Read Callback"="rsscope_FormatSearchNameReal64_ReadCallback.vi", "Write Callback"="rsscope_FormatSearchNameReal64_WriteCallback.vi", "Supported Models"="", "Instrument Options"="", "Flags"=0, "Help"="Defines the width of 
